vi "m10.wfg.test.vi"() -> ()   [LabVIEW 2012]
panel:
  in  "WF4 Par 1":dbl=2000.0
  in  "WF4 Par 0":dbl=4000.0
  in  "WF3 Par 0":dbl=2000.0
  in  "Dur (s)":dbl=0.5
  out "Waveform 4 FM":waveform(dbl)(graph)
  out "Waveform 3 PT":waveform(dbl)(graph)
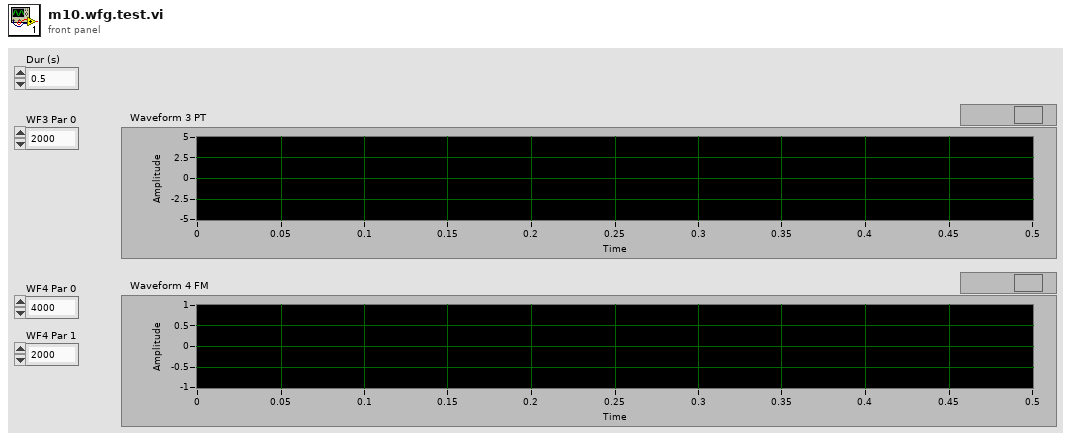
[diagram p1: front panel]
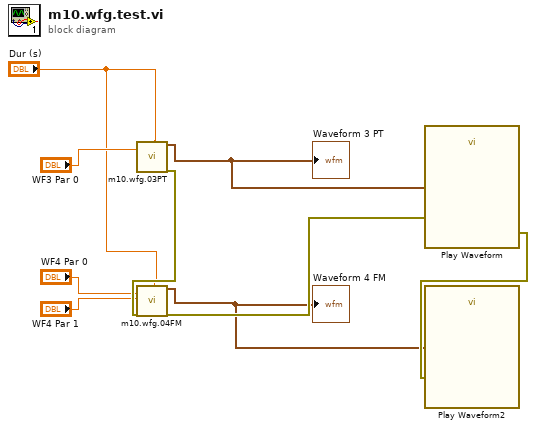
[diagram p0: block diagram]
diagram:
  n1 = call "m10.wfg.03PT.vi"("Param 0"="WF3 Par 0", "Duration (s)"="Dur (s)") -> ("Waveform Out"=w9:waveform(dbl), "error out"=w8:errorcluster)  [unwired: 16 in]
  "Waveform 3 PT" <- w9
  n2 = call "m10.wfg.04FM.vi"("Param 0"="WF4 Par 0", "Param 1"="WF4 Par 1", "error in (no error)"=w8, "Duration (s)"="Dur (s)") -> ("Waveform Out"=w1:waveform(dbl), "error out"=w2:errorcluster)  [unwired: 14 in]
  "Waveform 4 FM" <- w1
  n3 = call "Play Waveform"("Data"=w9, "error in"=w2) -> ("error out"=w3:errorcluster)  [unwired: 17 in]
  n4 = call "Play Waveform2"("Data"=w1, "error in"=w3) -> ()  [unwired: 17 in, 1 out]
